vi "ConvertJSON.vi"(11 "standard output":string) -> (1 "class":string, 2 "Most lik":cluster{"score":dbl, "class":string}[](array[cluster]), 3 "All Data":T1, 4 "score":dbl)   [LabVIEW 2019]
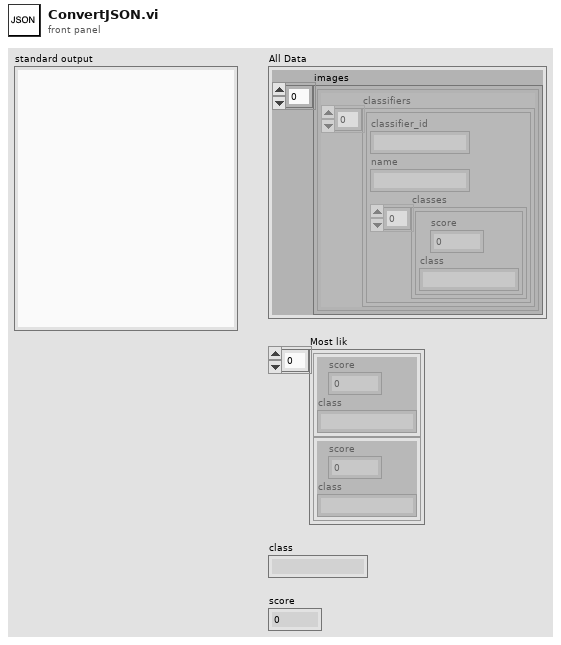
[diagram p1: front panel]
types:
  T1 = cluster{"images":cluster{"classifiers":cluster{"classifier_id":string, "name":string, "classes":cluster{"score":dbl, "class":string}[]}[]}[]}
  T2 = cluster{"classifiers":cluster{"classifier_id":string, "name":string, "classes":cluster{"score":dbl, "class":string}[]}[]}[]
  T3 = cluster{"classifier_id":string, "name":string, "classes":cluster{"score":dbl, "class":string}[]}[]
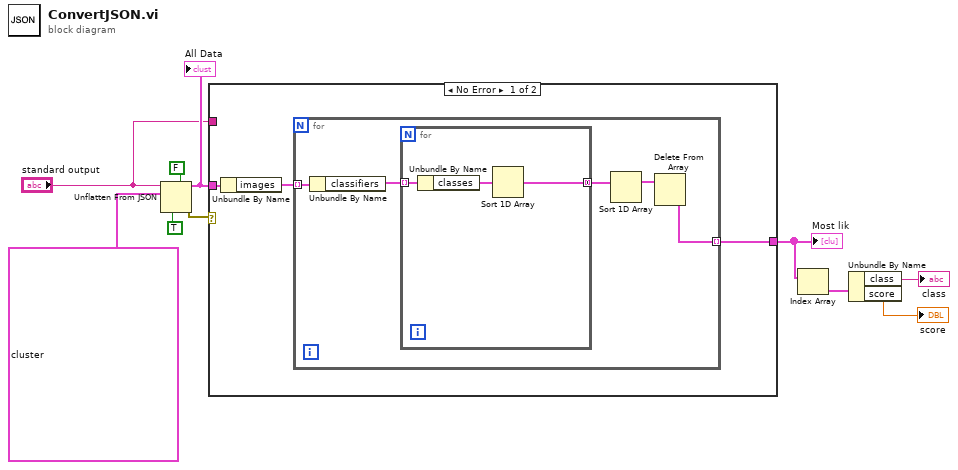
[diagram p0: block diagram]
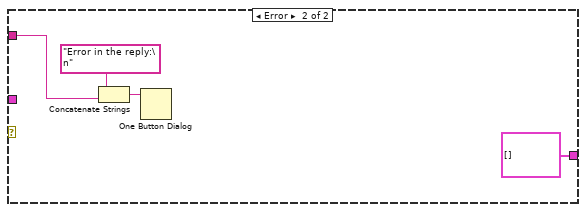
[diagram p2: hidden frame]
diagram:
  n1 = Unflatten From JSON(enable LabVIEW extensions? (T)=FALSE, JSON string="standard output", type and defaults=T1 {"images"=[{"classifiers"=[{"classifier_id"="", "name"="", "classes"=[{"score"=0.0, "class"=""}]}]}]}, default null elements? (F)=TRUE) -> (value=w6:T1, error out=w5:errorcluster)  [unwired: 3 in]
  "All Data" <- w6
  n2 = case shown="No Error" w5 {
    tunnel: w6 -> [w13 _]
    tunnel: [w11 cluster{"score":dbl, "class":string}[] []] -> w7
    tunnel: "standard output" -> [_ w23]
    frame No Error {
      n3 = Unbundle By Name(w13) -> ("images"=w12:T2)
      n4 = for {
        tunnel: w12 -> [w18] mode=indexing
        tunnel: [w15] -> w11 mode=indexing
        n5 = Unbundle By Name(w18) -> ("classifiers"=w17:T3)
        n6 = for {
          tunnel: w17 -> [w21] mode=indexing
          tunnel: [w19] -> w14 mode=concatenating
          n7 = Unbundle By Name(w21) -> ("classes"=w20:cluster{"score":dbl, "class":string}[])
          n8 = Sort 1D Array(array=w20) -> (sorted array=w19:cluster{"score":dbl, "class":string}[])
        }
        n9 = Sort 1D Array(array=w14) -> (sorted array=w16:cluster{"score":dbl, "class":string}[])
        n10 = Delete From Array(array=w16) -> (deleted portion=w15:cluster{"score":dbl, "class":string})  [unwired: 2 in, 1 out]
      }
    }
    frame Error {
      n11 = Concatenate Strings("Error in the reply:\n", w23) -> (w22:string)
      n12 = One Button Dialog(message=w22) -> ()  [unwired: 1 in, 1 out]
    }
  }
  "Most lik" <- w7
  n13 = Index Array(array=w7) -> (element=w8:cluster{"score":dbl, "class":string})  [unwired: 1 in]
  n14 = Unbundle By Name(w8) -> ("class"=→"class":string, "score"=→"score":dbl)
